vi "Send Parameter Message.vi"(8 "error in (no error)":errorcluster, 10 "ctlr queue":refnum<queue>, 11 "IA Test Parameters in":refnum<class "IA Test Parameters.lvclass">) -> (0 "error out":errorcluster)   [LabVIEW 2020]
uses:
  File Interfacing/Filename Structure.ctl
  Hardware/Actuators/Switches/Switch.lvclass
  Hardware/Actuators/Servos/Servo.lvclass
  Hardware/Sensors/Force Sensors/Force Sensor.lvclass
  Hardware/Sensors/Cameras/Camera.lvclass
  Controllers/Controller.lvclass
  Inflation Test/Parameter Class/IA Test Parameters.lvclass
  Controller Loop/Message and Data.ctl
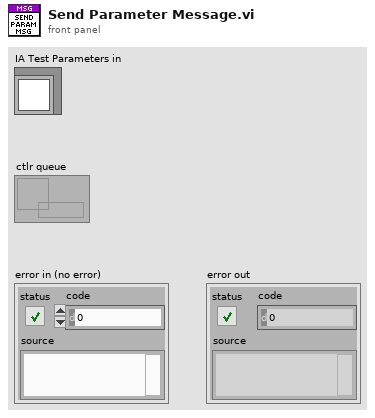
[diagram p1: front panel]
types:
  T1 = typedef "Message and Data.ctl" = cluster{"msg":string, "ia test param":refnum<class "IA Test Parameters.lvclass">, "controller type":refnum<class "Controller.lvclass">, "folder path":path, "file name":string, "file comments":string, "cam":refnum<class "Camera.lvclass">, "fs":refnum<class "Force Sensor.lvclass">, "servo":refnum<class "Servo.lvclass">, "switch":refnum<class "Switch.lvclass">, "filename struct":T2, "mm/pixel":dbl, "rectangle":T3}
  T2 = typedef "Filename Structure.ctl" = enum16{"<nameYYYYMMDDi>", "<name>"}
  T3 = typedef "IMAQ Rectangle" = cluster{"Left":i32, "Top":i32, "Right":i32, "Bottom":i32, "Rotation":dbl}
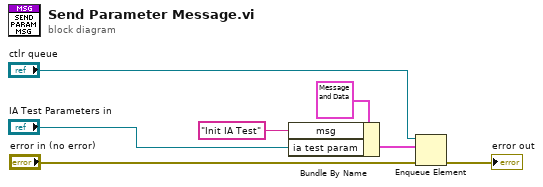
[diagram p0: block diagram]
diagram:
  n1 = Bundle By Name(cluster=T1 {"msg"="", "ia test param"=refnum, "controller type"=refnum, "folder path"=path "", "file name"="", "file comments"="", "cam"=refnum, "fs"=refnum, "servo"=refnum, "switch"=refnum, "filename struct"=enum."<nameYYYYMMDDi>", "mm/pixel"=0.0, "rectangle"={"Left"=0, "Top"=0, "Right"=0, "Bottom"=0, "Rotation"=0.0}} ("element"), "msg"="Init IA Test", "ia test param"="IA Test Parameters in") -> (w3:T1)
  n2 = Enqueue Element(queue="ctlr queue", element=w3, error in (no error)="error in (no error)") -> (error out=→"error out":errorcluster)  [unwired: 1 in, 2 out]
